vi "image.vi"() -> ()   [LabVIEW 2012]
uses:
  <vilib>/userdefined/High Color/IMAQdx.ctl
  <vilib>/vision/driver/NI_Vision_Acquisition_Software.lvlib
panel:
  in  "Blank Button":bool
  out "Image 2":T1(plugin-control)
  in  "IMAQdx Session":T2
  out "Image":T1(plugin-control)
  in  "Stop Button":bool
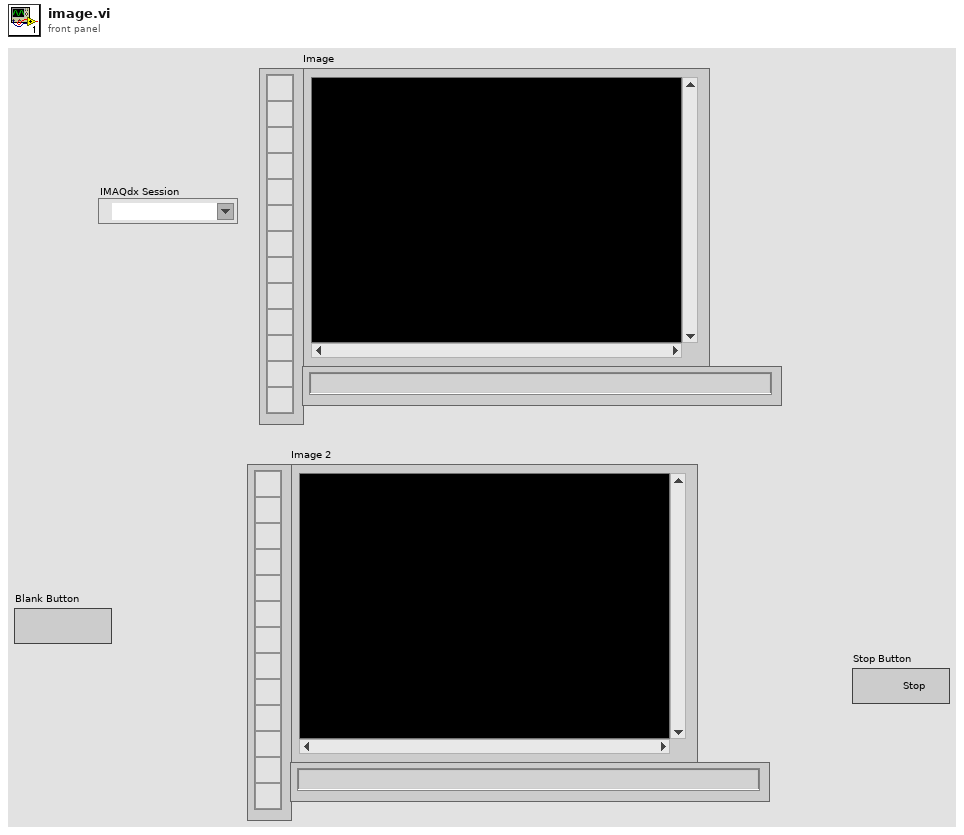
[diagram p1: front panel]
types:
  T1 = typedef "IMAQ Image.ctl" = refnum<image>
  T2 = typedef "IMAQdx.ctl" = refnum<k21>
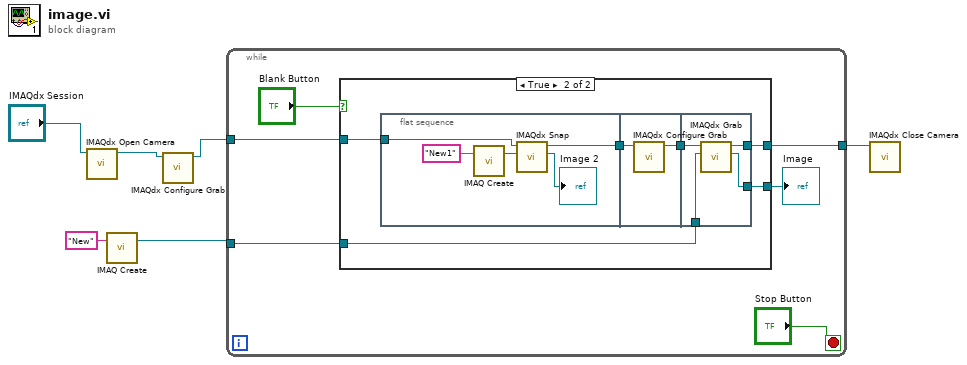
[diagram p0: block diagram]
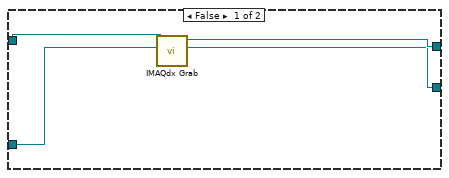
[diagram p2: hidden frame]
diagram:
  n1 = call <vilib>:"IMAQdx Open Camera.vi"("Session In"="IMAQdx Session") -> ("Session Out"=w2:T2)  [unwired: 9 in, 1 out]
  n2 = call "IMAQ Create"("Image Name"="New") -> ("New Image"=w4:T1)  [unwired: 4 in, 1 out]
  n3 = call <vilib>:"IMAQdx Configure Grab.vi"("Session In"=w2) -> ("Session Out"=w1:T2)  [unwired: 9 in, 1 out]
  n4 = while {
    tunnel: w4 -> [w9]
    tunnel: w1 -> [w10]
    tunnel: [w8] -> w3
    stop <- "Stop Button" stop-if-true
    n5 = case shown="True" "Blank Button" {
      tunnel: w10 -> [w15 w22]
      tunnel: w9 -> [w16 w19]
      tunnel: [w14 w18] -> w8
      tunnel: [w13 w17] -> w7
      frame False {
        n6 = call <vilib>:"IMAQdx Grab.vi"("Image In"=w16, "Session In"=w15) -> ("Image Out"=w13:T1, "Session Out"=w14:T2)  [unwired: 6 in, 2 out]
      }
      frame True {
        n7 = flat-sequence {
          tunnel: w22 -> [w24]
          tunnel: [w23] -> w21
          tunnel: w21 -> [w29]
          tunnel: [w28] -> w20
          tunnel: w20 -> [w33]
          tunnel: w19 -> [w32]
          tunnel: [w31] -> w18
          tunnel: [w30] -> w17
          frame #0 {
            n8 = call "IMAQ Create"("Image Name"="New1") -> ("New Image"=w25:T1)  [unwired: 4 in, 1 out]
            n9 = call <vilib>:"IMAQdx Snap.vi"("Image In"=w25, "Session In"=w24) -> ("Image Out"=→"Image 2":T1, "Session Out"=w23:T2)  [unwired: 7 in, 1 out]
          }
          frame #1 {
            n10 = call <vilib>:"IMAQdx Configure Grab.vi"("Session In"=w29) -> ("Session Out"=w28:T2)  [unwired: 9 in, 1 out]
          }
          frame #2 {
            n11 = call <vilib>:"IMAQdx Grab.vi"("Image In"=w32, "Session In"=w33) -> ("Image Out"=w30:T1, "Session Out"=w31:T2)  [unwired: 6 in, 2 out]
          }
        }
      }
    }
    "Image" <- w7
  }
  n12 = call <vilib>:"IMAQdx Close Camera.vi"("Session In"=w3) -> ()  [unwired: 10 in, 1 out]
